vi "Globals (private).vi"() -> ()   [LabVIEW 2015, in "SB SubVIs.lvlib"]
uses:
  SB SubVIs.lvlib
  Square/Square.lvclass
panel:
  out "Player List":string[](array[string])
  in  "Collisions":i32[](array[numeric])
  in  "Kills":i32[](array[numeric])
  in  "Generated":i32[](array[numeric])
  in  "Squares":i32[](array[numeric])
  in  "Round":i32
  in  "Winning":i32
  in  "Board Size":i32
  out "Players":refnum<class "Square.lvclass">[](array[class])
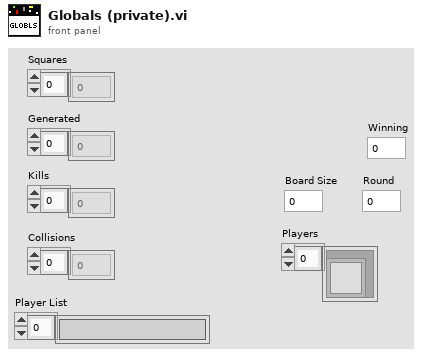
[diagram p1: front panel]
diagram:
